vi "Configure Setpoints Parameters.vi"(0 "VISA resource name":refnum<visa-resource-name>, 1 "Unit Address (1)":u8=1 min=1 max=254, 5 "Setpoint Rate Limit Value (0)":sgl min=0, 9 "Setpoint Ramp Units (0:Min)":u16(ring) items=["Min", "Hour", "Sec"], 11 "error in (no error)":errorcluster, 12 "Setpoint Trim Value (0)":sgl) -> (4 "VISA resource name out":refnum<visa-resource-name>, 15 "error out":errorcluster)   [LabVIEW 2010, in "Eurotherm 32xx Series.lvlib"]
doc: "This VI configure setpoints parameters."
uses:
  <instrlib>/Eurotherm 32xx Series/Eurotherm 32xx Series.lvlib
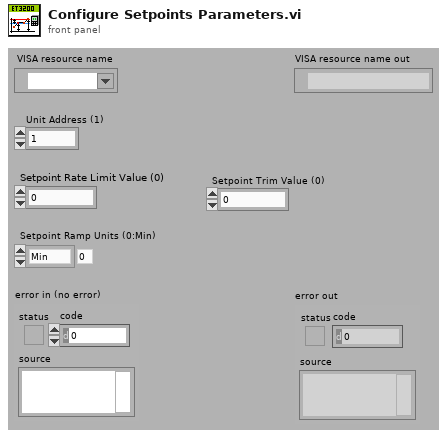
[diagram p1: front panel]
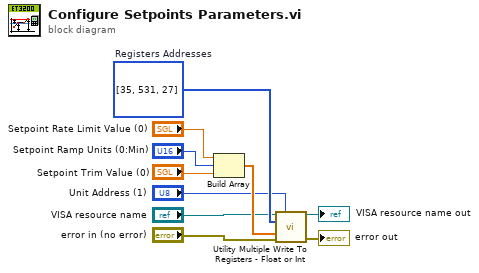
[diagram p0: block diagram]
diagram:
  w6 = u16[] [35, 531, 27]  # Registers Addresses
  n1 = Build Array("Setpoint Rate Limit Value (0)", "Setpoint Ramp Units (0:Min)", "Setpoint Trim Value (0)") -> (w7:sgl[])
  n2 = call <instrlib>:"Utility Multiple Write To Registers - Float or Int.vi"("VISA resource name"="VISA resource name", "Unit Address (1)"="Unit Address (1)", "Registers Addresses (0)"=w6, "Data (0)"=w7, "error in (no error)"="error in (no error)") -> ("VISA resource name out"=→"VISA resource name out":refnum<visa-resource-name>, "error out"=→"error out":errorcluster)  [unwired: 9 in]
